vi "Cowl_Hardware_Globals.vi"() -> ()   [LabVIEW 2020]
panel:
  in  "Cowl Motor":string="Cowl Motor"
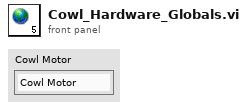
[diagram p1: front panel]
diagram:
